vi "Solve Linear Equations By Cholesky.vi"(3 "Known Vector":dbl[](array[numeric]) format="%.2f", 4 "Input Matrix":T1) -> (0 "error":i32, 1 "Solution Vector":dbl[](array[numeric]) format="%.2f")   [LabVIEW 2018, in "NI_AALBase.lvlib"]
doc: "Solves a real linear system AX=Y using Cholesky factorization."
uses:
  NI_AALBase.lvlib
  RealMatrix.ctl
  <resource>/lvanlys.dll
  NI_Matrix.lvlib
panel:
  # "Solve Positive Definite Linear Equations"
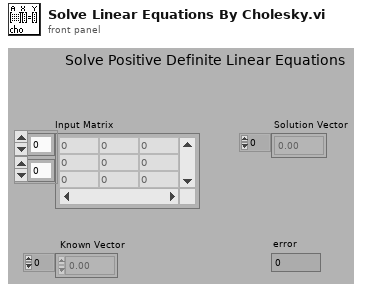
[diagram p1: front panel]
types:
  T1 = typedef "NI_Matrix.lvlib/RealMatrix.ctl" = dbl[][]
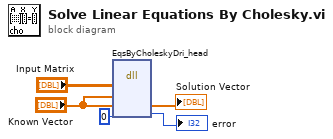
[diagram p0: block diagram]
diagram:
  n1 = dll-call lib="C:/Program Files (x86)/National Instruments/LabVIEW 2018/resource/lvanlys.*" fn="EqsByCholeskyDri_head"("Input Matrix"="Input Matrix", "Known Vector"="Known Vector", "Known Vector"="Known Vector", 0) -> ("Known Vector"=→"Solution Vector":dbl[], →"error":i32)  [unwired: 6 in, 2 out]
